vi "SEK2020v1SubVIGiro.vi"(6 "ANGULO":sgl, 8 "NXT/EV3":T1) -> (2 "NXT/EV3 2":T1)   [LabVIEW 2016]
uses:
  <vilib>/NXT/Subs/LVHSConnector.ctl
  <vilib>/NXT/LegoClasses/BrickReference/BrickReference.lvclass
  <vilib>/NXT/Block Support/NXT_OutputPort.ctl
  <vilib>/NXT/Block Support/NXT_InputPort.ctl
  <vilib>/NXT/Dual Mode Library/Sensors/EV3_Gyro_Angle.vi
  <vilib>/NXT/Dual Mode Library/Waits/Wait_Num.vi
  <vilib>/NXT/Dual Mode Library/Sensors/EV3_Gyro_Reset.vi
  <vilib>/NXT/NXTIO Xnodes/NXTIONodeSubVIs/NXTMoveMotors.vi
  <vilib>/NXT/NXTIO Xnodes/NXTIONodeSubVIs/NXTStopMotors.vi
  <vilib>/NXT/NXTIO Xnodes/AddressXNode/NXTIOAddress.xnode
  <vilib>/NXT/NXTIO Xnodes/NXTIOXNode/NXTIO.xnode
panel:
  out "NXT/EV3 3":T1
  in  "Kp 2":sgl
  in  "Ki 2":sgl
  in  "Kd 2":sgl
  in  "Kd":sgl
  in  "Ki":sgl
  in  "Kp":sgl
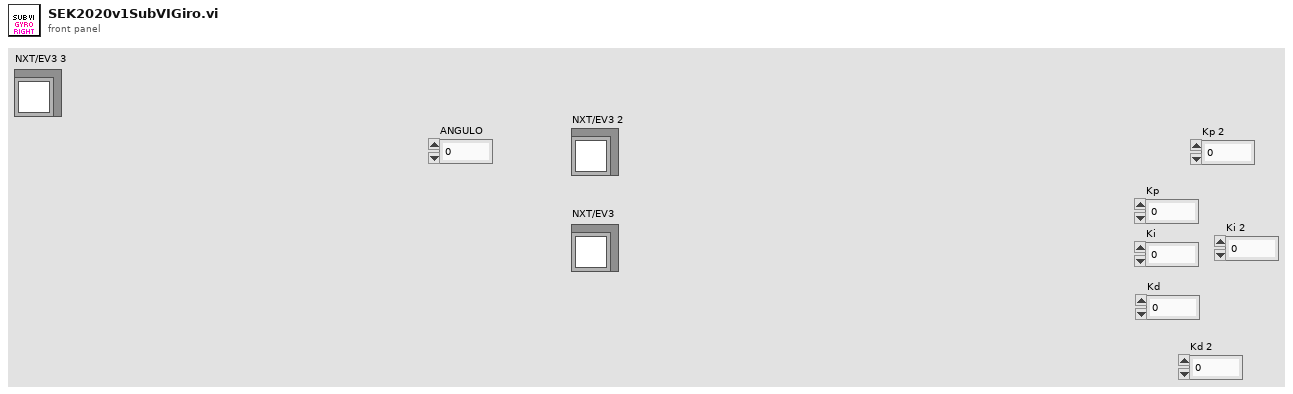
[diagram p1: front panel]
types:
  T1 = typedef "LVHSConnector.ctl" = refnum<class "BrickReference.lvclass">
  T2 = typedef "NXT_InputPort.ctl" = u32
  T3 = typedef "NXT_OutputPort.ctl" = u8
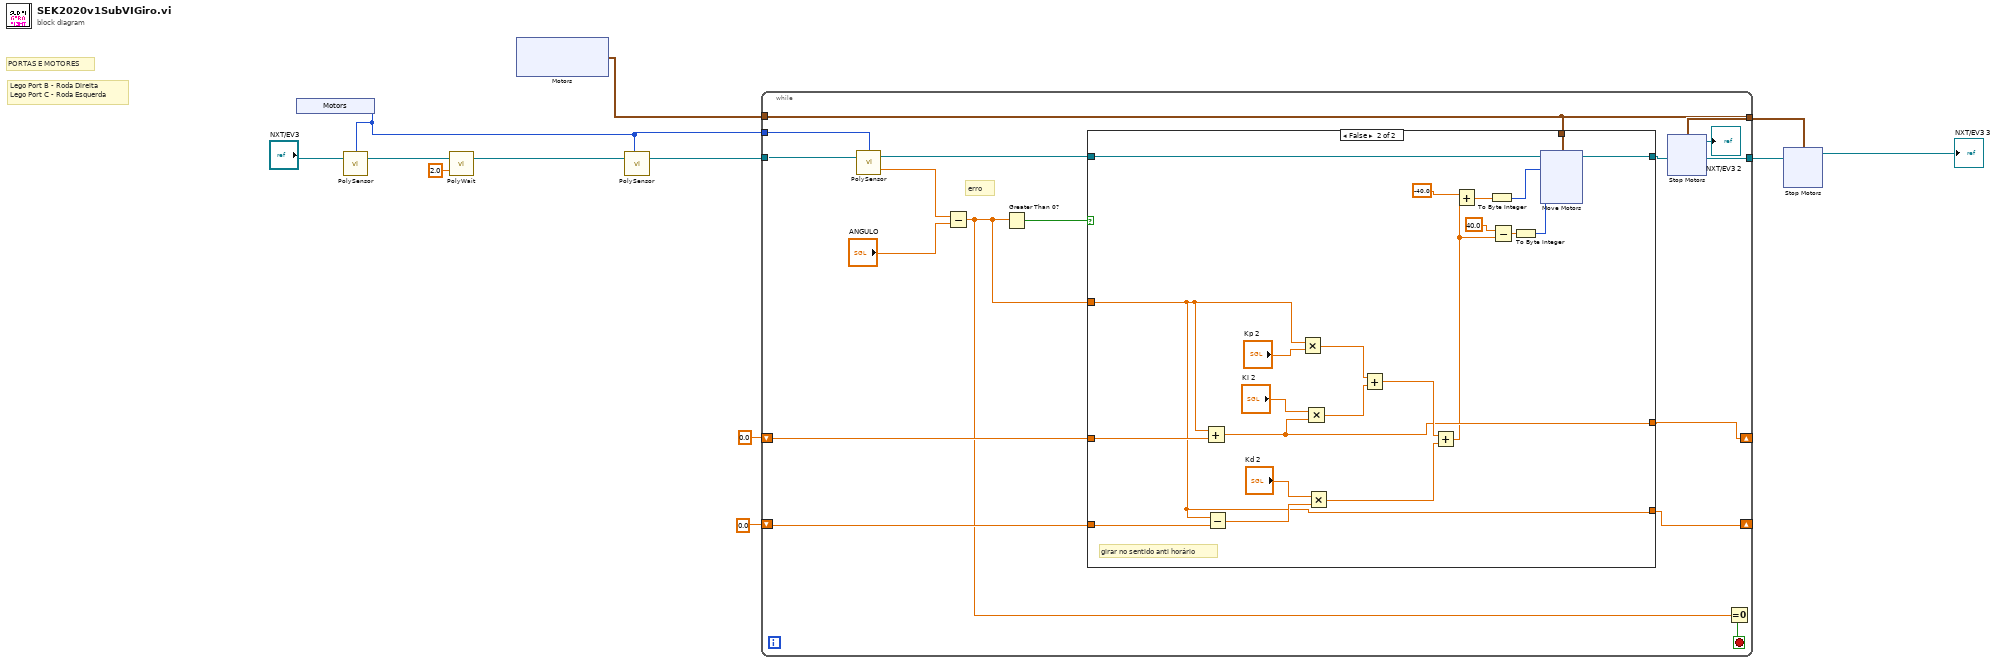
[diagram p0: block diagram]
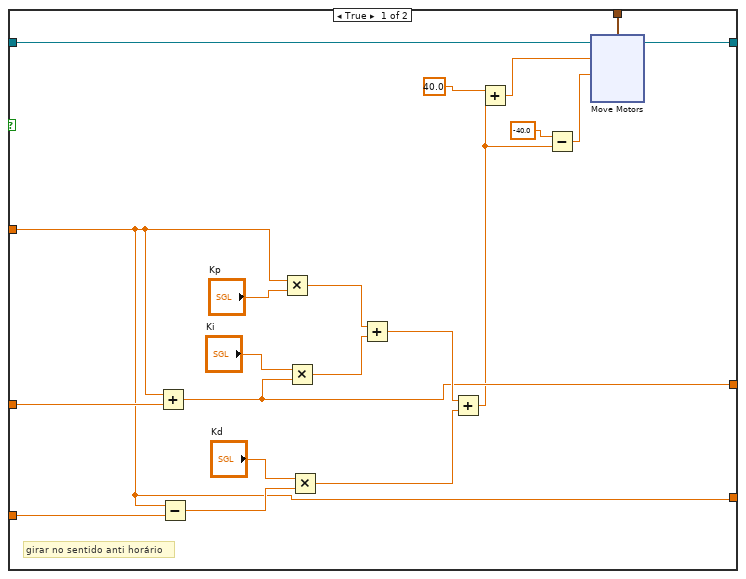
[diagram p2: hidden frame]
diagram:
  # "Lego Port B - Roda Direita\nLego Port C - Roda Esquerda"
  # "PORTAS E MOTORES"
  n1 = xnode "Motors"() -> ("Sensor"=w2:T2)
  n2 = call-poly <vilib>:"PolySensor.vi"("NXT/EV3"="NXT/EV3", "Port (Port 1)"=w2) -> ("NXT/EV3"=w4:T1)  [unwired: 1 in, 1 out]
  n3 = call-poly <vilib>:"PolyWait.vi"("Time (1 sec)"=sgl 2.0, "NXT/EV3"=w4) -> ("NXT/EV3"=w3:T1)  [unwired: 2 in]
  n4 = xnode "Motors"() -> ("Motor"=w13:cluster{"Port":T3, "Port":T3})
  n5 = call-poly <vilib>:"PolySensor.vi"("NXT/EV3"=w3, "Port (Port 1)"=w2) -> ("NXT/EV3"=w12:T1)  [unwired: 2 in]
  n6 = while {
    tunnel: w13 -> [w20]
    tunnel: w2 -> [w24]
    tunnel: [w20] -> w7
    tunnel: w12 -> [w26]
    shift-right: [w17] -> _
    shift-left: 0.0 -> [w19]
    shift-right: [w16] -> _
    shift-left: 0.0 -> [w18]
    tunnel: [w15] -> w8
    stop <- w27 stop-if-true
    # "erro"
    n7 = call-poly <vilib>:"PolySensor.vi"("NXT/EV3"=w26, "Port (Port 1)"=w24) -> ("Degrees"=w25:sgl, "NXT/EV3"=w21:T1)  [unwired: 1 in]
    n8 = Subtract(x=w25, y="ANGULO") -> (x-y=w14:sgl)
    n9 = Greater Than 0?(x=w14) -> (x > 0?=w22:bool)
    n10 = case shown="False" w22 {
      tunnel: w21 -> [w34 w64]
      tunnel: w14 -> [w35 w65]
      tunnel: w20 -> [w39 w69]
      tunnel: w19 -> [w38 w68]
      tunnel: w18 -> [w37 w67]
      tunnel: [w36 w66] -> w17
      tunnel: [w35 w65] -> w16
      tunnel: [w28 w60] -> w15
      frame True {
        # "girar no sentido anti horário"
        n11 = Add(x=w35, y=w38) -> (x+y=w36:dbl)
        n12 = Subtract(x=w35, y=w37) -> (x-y=w42:dbl)
        n13 = Multiply(x=w35, y="Kp") -> (x*y=w45:sgl)
        n14 = Multiply(x="Ki", y=w36) -> (x*y=w44:dbl)
        n15 = Multiply(x="Kd", y=w42) -> (x*y=w41:dbl)
        n16 = Add(x=w45, y=w44) -> (x+y=w40:dbl)
        n17 = Add(x=w40, y=w41) -> (x+y=w30:dbl)
        n18 = Add(x=40.0, y=w30) -> (x+y=w32:dbl)
        n19 = Subtract(x=-40.0, y=w30) -> (x-y=w29:dbl)
        n20 = xnode "Move Motors"("Power/Speed 2"=w29, "Power/Speed 1"=w32, "Motors"=w39, "NXT/EV3"=w34) -> ("NXT/EV3"=w28:T1)
      }
      frame False {
        # "girar no sentido anti horário"
        n21 = Add(x=w65, y=w68) -> (x+y=w66:dbl)
        n22 = Subtract(x=w65, y=w67) -> (x-y=w72:dbl)
        n23 = Multiply(x=w65, y="Kp 2") -> (x*y=w75:sgl)
        n24 = Multiply(x="Ki 2", y=w66) -> (x*y=w74:dbl)
        n25 = Multiply(x="Kd 2", y=w72) -> (x*y=w71:dbl)
        n26 = Add(x=w75, y=w74) -> (x+y=w70:dbl)
        n27 = Add(x=w70, y=w71) -> (x+y=w61:dbl)
        n28 = Add(x=-40.0, y=w61) -> (x+y=w58:dbl)
        n29 = To Byte Integer(number=w58) -> (8bit integer=w59:i8)
        n30 = Subtract(x=40.0, y=w61) -> (x-y=w57:dbl)
        n31 = To Byte Integer(number=w57) -> (8bit integer=w56:i8)
        n32 = xnode "Move Motors"("Power/Speed 2"=w56, "Power/Speed 1"=w59, "Motors"=w69, "NXT/EV3"=w64) -> ("NXT/EV3"=w60:T1)
      }
    }
    n33 = Equal To 0?(x=w14) -> (x = 0?=w27:bool)
  }
  n34 = xnode "Stop Motors"("Motors"=w7) -> ("NXT/EV3"=→"NXT/EV3 2":T1)  [unwired: 1 in]
  n35 = xnode "Stop Motors"("Motors"=w7, "NXT/EV3"=w8) -> ("NXT/EV3"=→"NXT/EV3 3":T1)
